vi "SCPI Version Query.vi"(8 "error in (no error)":errorcluster, 11 "VISA resource name":refnum<visa-resource-name>) -> (0 "error out":errorcluster, 2 "Version":string, 3 "VISA resource name out":refnum<visa-resource-name>)   [LabVIEW 2018, in "XP Power PLS600.lvlib"]
doc: "Queries the version of the SCPI specification which is supported by the instrument."
uses:
  XP Power PLS600.lvlib
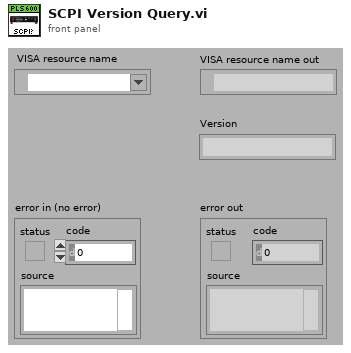
[diagram p1: front panel]
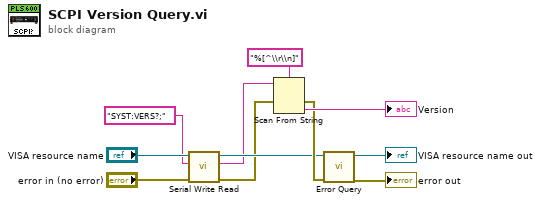
[diagram p0: block diagram]
diagram:
  n1 = call "Serial Write Read.vi"("error in (no error)"="error in (no error)", "Write Buffer"="SYST:VERS?;", "VISA resource name"="VISA resource name") -> ("error out"=w2:errorcluster, "Read Buffer"=w3:string, "VISA resource name out"=w4:refnum<visa-resource-name>)  [unwired: 6 in]
  n2 = Scan From String(format string="%[^\\r\\n]", input string=w3, error in=w2) -> (error out=w7:errorcluster, output 1=→"Version":string)  [unwired: 2 in, 2 out]
  n3 = call "Error Query.vi"("error in (no error)"=w7, "VISA resource name"=w4) -> ("error out"=→"error out":errorcluster, "VISA resource name out"=→"VISA resource name out":refnum<visa-resource-name>)  [unwired: 6 in, 2 out]
